vi "Leds.vi"() -> ()   [LabVIEW 2018]
panel:
  in  "millisecond multiple":u32=100
  out "L4":bool
  out "L3":bool
  out "L2":bool
  out "L1":bool
  in  "stop":bool
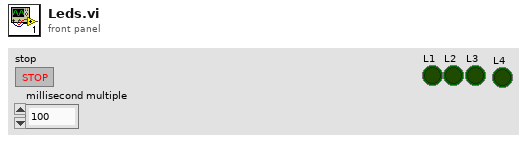
[diagram p1: front panel]
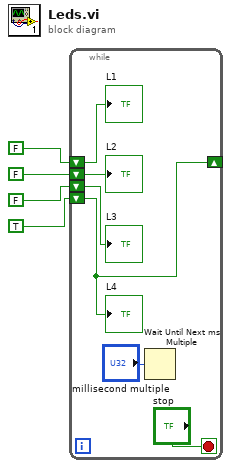
[diagram p0: block diagram]
diagram:
  n1 = while {
    shift-right: [w5] -> _
    shift-left: FALSE -> [w8]
    shift-left: FALSE -> [w7]
    shift-left: FALSE -> [w6]
    shift-left: TRUE -> [w5]
    stop <- "stop" stop-if-true
    n2 = Wait Until Next ms Multiple(millisecond multiple="millisecond multiple") -> ()  [unwired: 1 out]
    "L1" <- w8
    "L2" <- w7
    "L3" <- w6
    "L4" <- w5
  }
